vi "tableCleanerItem.vi"(8 "error in (no error)":errorcluster, 9 "storageSheets":T1, 10 "Table in":refnum<vi>, 11 "reference in":refnum<class "Project Panels.lvclass">) -> (0 "error out":errorcluster, 3 "reference out":refnum<class "Project Panels.lvclass">)   [LabVIEW 2015, in "Project Panels.lvclass"]
uses:
  Project Panels.lvclass
  SYS/Items Controller_llb/storageSheets.ctl
  SYS/Items Controller_llb/Items Controller.lvclass
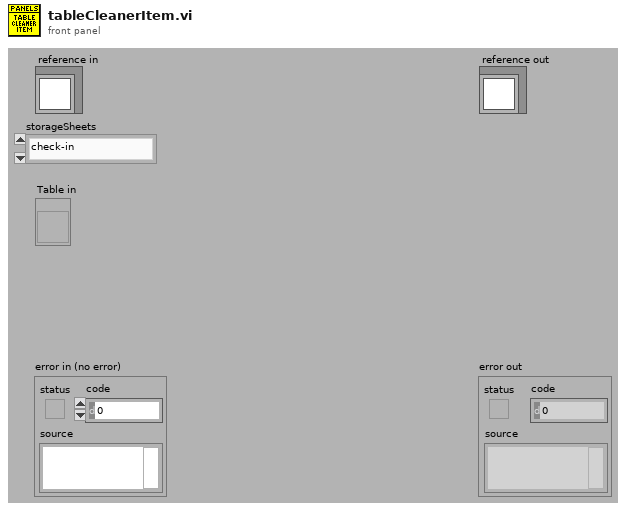
[diagram p1: front panel]
types:
  T1 = typedef "Items Controller.lvclass/storageSheets.ctl" = enum16{"check-in", "check-out", "storage"}
  T2 = enum16{"User-specified Font", "Application Font", "System Font", "Dialog Font"}
  T3 = cluster{"Font Name:":string, "Size":i16, "Strikeout?":bool, "Italic?":bool, "Underline?":bool, "Outline?":bool, "Shadow?":bool, "Bold?":bool}
  T4 = typedef "Project Panels.lvclass/ObjectAttributesRef.ctl" = refnum<data-value>
  T5 = typedef "Project Panels.lvclass/ObjectAttributes.ctl" = cluster{"MyAttribute":dbl, "device_controller_ref":refnum<class "Devices Controller.lvclass">, "file_controller_ref":refnum<class "File Controller.lvclass">, "item_controller_ref":refnum<class "Items Controller.lvclass">, "item_tables":cluster{"checkIN":string[][], "checkOUT":string[][], "storage":string[][]}, "quickbook_table":cluster{"notes":string[][]}, "notification_controller_ref":refnum<class "Notification Controller.lvclass">, "partstracking_controller_ref":refnum<class "PartsTracking Controller.lvclass">, "product_tables":cluster{"k4b2":string[][], "fitmate":string[][], "RMR":string[][], "CPET":string[][], "BP":string[][], "PP":string[][], "k5":string[][], "bb-pft":string[][]}, "rowsColour":u32[], "low_resolution?":bool, "run_python?":bool}
  T6 = cluster{"left":i16, "top":i16, "right":i16, "bottom":i16}
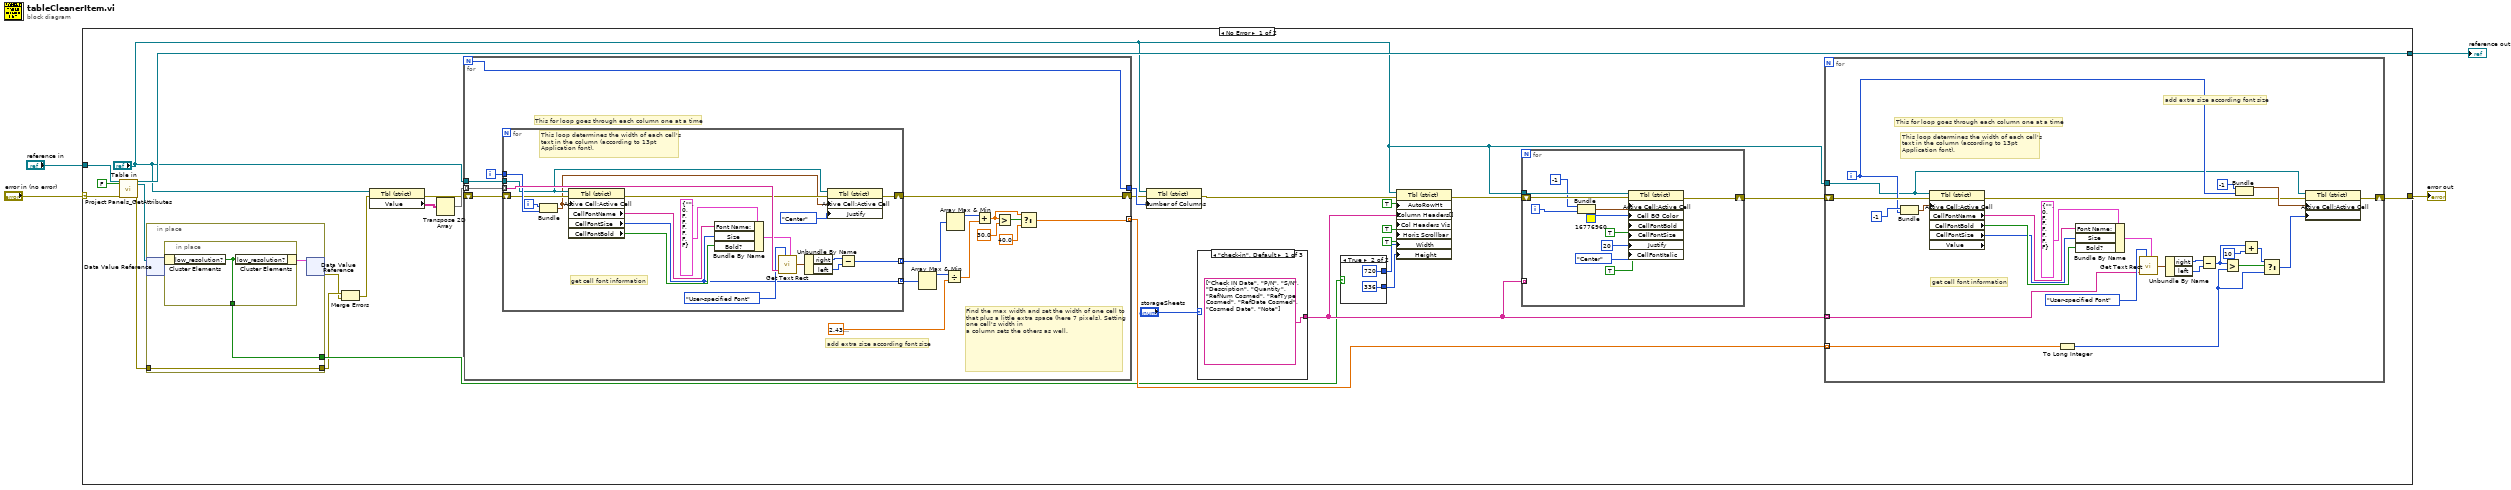
[diagram p0: block diagram]
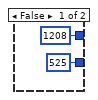
[diagram p2: hidden frame]
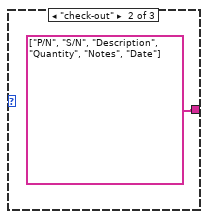
[diagram p3: hidden frame]
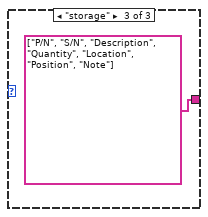
[diagram p4: hidden frame]
diagram:
  n1 = case shown="No Error" "error in (no error)" {
    selector: "error in (no error)" -> [w30 w119]
    tunnel: [w17 w119] -> w3
    tunnel: [w29 w118] -> w1
    tunnel: "reference in" -> [w32 w118]
    frame No Error {
      n2 = call "Project Panels_GetAttributes.vi"("reference in"=w32, "return data? (T)"=FALSE, "error in (no error)"=w30) -> ("reference out"=w29:refnum<class "Project Panels.lvclass">, "attributes ref"=w10:T4, "error out"=w8:errorcluster)  [unwired: 13 in, 1 out]
      n3 = in-place {
        in-place-border: w8 -> [w34]
        in-place-border: [w34] -> w7
        in-place-border: [w33] -> w9
        n4 = in-place-dvr #1(w10) -> (w35:T5)  [unwired: 1 out]
        n5 = in-place {
          in-place-border: [w37] -> w33
          n6 = in-place-cluster #2(w35) -> ("low_resolution?"=w37:bool)
          n7 = in-place-cluster #2("low_resolution?"=w37) -> (w36:T5)
        }
        n8 = in-place-dvr #1(w36) -> (w6:errorcluster)  [unwired: 1 out]
      }
      n9 = Merge Errors(w7, w6) -> (w5:errorcluster)
      n10 = property on="Property Node" class="Tbl (strict)"(reference="Table in", error in=w5) -> (error out=w24:errorcluster, "Value"=w25:string[][])  [unwired: 1 out]
      n11 = Transpose 2D Array(2D array=w25) -> (transposed array=w26:string[][])
      n12 = for {
        N -> [w90]
        tunnel: w26 -> [w98] mode=indexing
        tunnel: [w90] -> w28
        tunnel: "Table in" -> [w89]
        shift-right: [w82] -> w27
        shift-left: w24 -> [w88]
        tunnel: [w83] -> w11 mode=indexing
        i -> [w96]
        # "add extra size according font size"
        # "Find the max width and set the width of one cell to that plus a little extra space (here 7 pixels). Setting one cell's width in\na column sets the others as well."
        # "This for loop goes through each column one at a time"
        n13 = for {
          tunnel: w98 -> [w117] mode=indexing
          tunnel: [w113] -> w97 mode=indexing
          tunnel: w96 -> [w108]
          tunnel: [w105] -> w94 mode=indexing
          tunnel: w89 -> [w100]
          shift-right: [w102] -> w82
          shift-left: w88 -> [w104]
          i -> [w107]
          # "get cell font information"
          # "This loop determines the width of each cell's\ntext in the column (according to 13pt\nApplication font)."
          n14 = Bundle(w107, w108) -> (w99:cluster{i32, i32})  [unwired: 1 in]
          n15 = property on="Property Node" class="Tbl (strict)"(reference=w100, error in=w104, "Active Cell:Active Cell"=w99) -> (error out=w103:errorcluster, "CellFontName"=w112:string, "CellFontSize"=w105:u32, "CellFontBold"=w111:bool)  [unwired: 1 out]
          n16 = Bundle By Name(cluster=T3 {"Font Name:"="", "Size"=0, "Strikeout?"=FALSE, "Italic?"=FALSE, "Underline?"=FALSE, "Outline?"=FALSE, "Shadow?"=FALSE, "Bold?"=FALSE} ("[user-specified font]"), "Font Name:"=w112, "Size"=w105, "Bold?"=w111) -> (w109:T3)
          n17 = call <vilib>:"Get Text Rect.vi"("desired font(Application)"=T2."User-specified Font", "text"=w117, "[user-specified font]"=w109) -> ("rect"=w116:T6)  [unwired: 6 in]
          n18 = Unbundle By Name(w116) -> ("right"=w115:i16, "left"=w114:i16)
          n19 = property on="Property Node" class="Tbl (strict)"(reference=w100, error in=w103, "Active Cell:Active Cell"=w99, "Justify"=enum16{"Left", "Center", "Right"}."Center" ("Active Cell:Cell Justification")) -> (error out=w102:errorcluster)  [unwired: 1 out]
          n20 = Subtract(x=w115, y=w114) -> (x-y=w113:i16)
        }
        n21 = Array Max & Min(array=w94) -> (max value=w93:u32)  [unwired: 3 out]
        n22 = Divide(x=w93, y=sgl 2.43) -> (x/y=w91:sgl)
        n23 = Array Max & Min(array=w97) -> (max value=w95:i16)  [unwired: 3 out]
        n24 = Add(x=w95, y=w91) -> (x+y=w84:sgl)
        n25 = Greater?(x=w84, y=sgl 30.0) -> (0:w86:bool)
        n26 = Select(t=w84, s=w86, f=sgl 40.0 ("y")) -> (s? t:f=w83:sgl)
      }
      n27 = property on="Property Node" class="Tbl (strict)"(reference="Table in", error in=w27, "Number of Columns"=w28) -> (error out=w18:errorcluster)  [unwired: 1 out]
      n28 = case shown="\"check-in\", Default" "storageSheets" {
        tunnel: [string[] ["Check IN Date", "P/N", "S/N", "Description", "Quantity", "RefNum Cosmed", "RefType Cosmed", "RefDate Cosmed", "Cosmed Date", "Note"] ("Column Header Strings[]") string[] ["P/N", "S/N", "Description", "Quantity", "Notes", "Date"] ("Column Header Strings[]") string[] ["P/N", "S/N", "Description", "Quantity", "Location", "Position", "Note"] ("Column Header Strings[]")] -> w13
        frame "check-in", Default {
        }
        frame "check-out" {
        }
        frame "storage" {
        }
      }
      n29 = case shown="True" w9 {
        tunnel: [u32 1208 ("Size:Width") u32 720 ("Size:Width")] -> w20
        tunnel: [u32 525 ("Size:Width") u32 336 ("Size:Width")] -> w19
        frame False {
        }
        frame True {
        }
      }
      n30 = property on="Property Node" class="Tbl (strict)"(reference="Table in", error in=w18, "AutoRowHt"=TRUE ("Autosizing Row Height"), "Column Headers[]"=w13, "Col Headers Vis"=TRUE ("Visible Items:Column Headers Visible"), "Horiz Scrollbar"=TRUE ("Visible Items:Horizontal Scrollbar Visible"), "Width"=w20, "Height"=w19) -> (error out=w16:errorcluster)  [unwired: 1 out]
      n31 = for {
        tunnel: "Table in" -> [w76]
        tunnel: w13 -> [_] mode=indexing
        shift-right: [w77] -> w15
        shift-left: w16 -> [w78]
        i -> [w74]
        n32 = Bundle("index"=-1, w74) -> (w75:cluster{"index":i32, i32})  [unwired: 1 in]
        n33 = property on="Property Node" class="Tbl (strict)"(reference=w76, error in=w78, "Active Cell:Active Cell"=w75, "Cell BG Color"=u32 16776960, "CellFontBold"=TRUE ("Active Cell:Cell Font:Bold"), "CellFontSize"=u32 20 ("Active Cell:Cell Font:Size"), "Justify"=enum16{"Left", "Center", "Right"}."Center" ("Active Cell:Cell Justification"), "CellFontItalic"=TRUE ("Active Cell:Cell Font:Italic")) -> (error out=w77:errorcluster)  [unwired: 1 out]
      }
      n34 = for {
        tunnel: "Table in" -> [w47]
        shift-right: [w65] -> w17
        shift-left: w15 -> [w64]
        tunnel: w13 -> [w45] mode=indexing
        tunnel: w11 -> [w43] mode=indexing
        i -> [w53]
        # "get cell font information"
        # "This loop determines the width of each cell's\ntext in the column (according to 13pt\nApplication font)."
        # "add extra size according font size"
        # "This for loop goes through each column one at a time"
        n35 = Bundle("index"=-1, w53) -> (w52:cluster{"index":i32, i32})  [unwired: 1 in]
        n36 = property on="Property Node" class="Tbl (strict)" props=["Active Cell:Active Cell", "CellFontName", "CellFontBold", "CellFontSize", "Value"](reference=w47, error in=w64, "Active Cell:Active Cell"=w52) -> (error out=w44:errorcluster, "CellFontName"=w59:string, "CellFontBold"=w58:bool, "CellFontSize"=w46:u32)  [unwired: 2 out]
        n37 = To Long Integer(number=w43) -> (32bit integer=w42:i32)
        n38 = Bundle By Name(cluster=T3 {"Font Name:"="", "Size"=0, "Strikeout?"=FALSE, "Italic?"=FALSE, "Underline?"=FALSE, "Outline?"=FALSE, "Shadow?"=FALSE, "Bold?"=FALSE} ("[user-specified font]"), "Font Name:"=w59, "Size"=w46, "Bold?"=w58) -> (w56:T3)
        n39 = call <vilib>:"Get Text Rect.vi"("desired font(Application)"=T2."User-specified Font", "text"=w45, "[user-specified font]"=w56) -> ("rect"=w62:T6)  [unwired: 6 in]
        n40 = Unbundle By Name(w62) -> ("right"=w61:i16, "left"=w60:i16)
        n41 = Subtract(x=w61, y=w60) -> (x-y=w50:i16)
        n42 = Greater?(x=w50, y=w42) -> (0:w51:bool)
        n43 = Bundle(-1, w53) -> (w66:cluster{i32, i32})  [unwired: 1 in]
        n44 = Add(x=w50, y=i16 10) -> (x+y=w48:i16)
        n45 = Select(t=w48, s=w51, f=w42) -> (s? t:f=w63:i32)
        n46 = property on="Property Node" class="Tbl (strict)"(reference=w47, error in=w44, "Active Cell:Active Cell"=w66, "Active Cell:Cell Size:Width"=w63) -> (error out=w65:errorcluster)  [unwired: 1 out]
      }
    }
    frame Error {
    }
  }
  "error out" <- w3
  "reference out" <- w1
